vi "NI VeriStand - Stop Workspace File.vi"(8 "error in (no error)":errorcluster, 10 "Password (\"\")":string, 11 "WorkspaceManager in":T1) -> (0 "error out":errorcluster, 3 "WorkspaceManager out":T1)   [LabVIEW 2020, in "NI_VS Workspace ExecutionAPI.lvlib"]
doc: "Stops the workspace file that currently is running."
uses:
  <vilib>/NI VeriStand/Execution/Workspace/NI_VS Workspace ExecutionAPI.lvlib
  <vilib>/NI VeriStand/Execution/Workspace/WorkspaceAPI.ctl
  NationalInstruments.VeriStand.ClientAPI
panel:
  # "This VI has been deprecated in favor of NI VeriStand - Disconnect from System.vi."
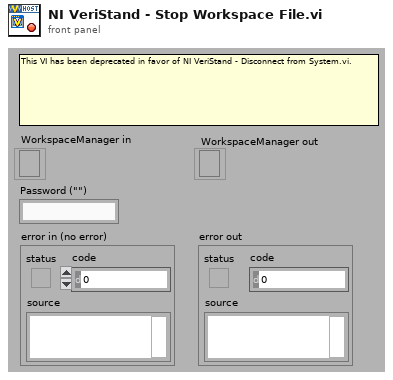
[diagram p1: front panel]
types:
  T1 = typedef "NI_VS Workspace ExecutionAPI.lvlib/WorkspaceAPI.ctl" = refnum<k24>
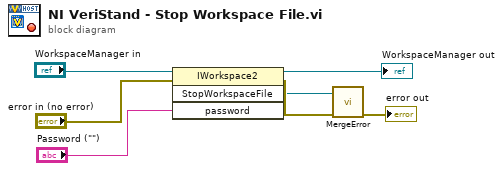
[diagram p0: block diagram]
diagram:
  n1 = invoke class="IWorkspace2" method="StopWorkspaceFile"(reference="WorkspaceManager in", error in="error in (no error)", "password"="Password (\"\")") -> (reference out=→"WorkspaceManager out":T1, error out=w5:errorcluster, "StopWorkspaceFile"=w4:refnum<k24>)  [unwired: 1 in, 1 out]
  n2 = call <vilib>:"MergeError.vi"("error in (no error)"=w5, "Error"=w4) -> ("error out"=→"error out":errorcluster)  [unwired: 9 out]
